vi "Sel UnSel Highlight.vi"(8 "error in (no error)":errorcluster, 10 "Check All? (T)":bool=TRUE, 11 "Methods ListCtrl":refnum<vi>) -> (0 "error out":errorcluster, 3 "Methods ListCtrl 2":refnum<vi>)   [LabVIEW 2020, in "WebServiceImporter.lvlib" / "Main Panel.lvlib" / "Select Methods.lvlib"]
uses:
  <vilib>/Platform/WebService/Main Panel/Pages/Select Methods/Select Methods.lvlib
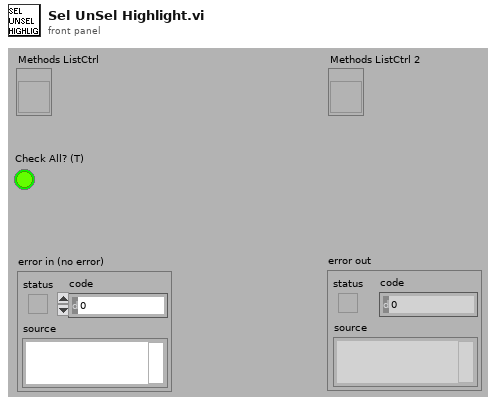
[diagram p1: front panel]
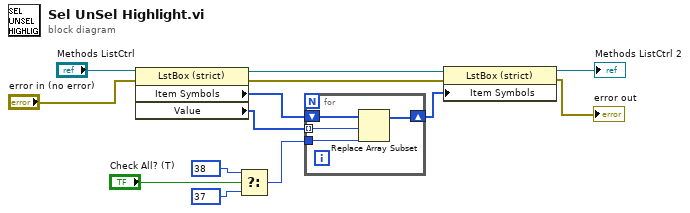
[diagram p0: block diagram]
diagram:
  n1 = property class="LstBox (strict)"(reference="Methods ListCtrl", error in="error in (no error)") -> (reference out=w5:refnum<vi>, error out=w4:errorcluster, "Item Symbols"=w7:i32[], "Value"=w8:i32[])
  n2 = Select(t=38, s="Check All? (T)", f=37) -> (s? t:f=w6:i32)
  n3 = for {
    tunnel: w8 -> [w16] mode=indexing
    shift-right: [w14] -> w3
    shift-left: w7 -> [w17]
    tunnel: w6 -> [w15]
    n4 = Replace Array Subset(array=w17, new element=w15, index=w16) -> (w14:i32[])
  }
  n5 = property class="LstBox (strict)"(reference=w5, error in=w4, "Item Symbols"=w3) -> (reference out=→"Methods ListCtrl 2":refnum<vi>, error out=→"error out":errorcluster)
